vi "record_tsv_LCWFM.vi"(7 "record_on":bool=TRUE, 8 "value_array":dbl[](array[numeric])=[0.0], 10 "time":timestamp, 11 "file_name":string="record") -> (0 "status":bool)   [LabVIEW 2019]
uses:
  <vilib>/Utility/file.llb/Write Delimited Spreadsheet (string).vi
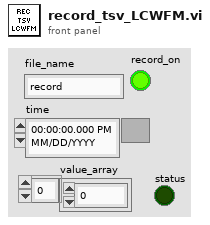
[diagram p1: front panel]
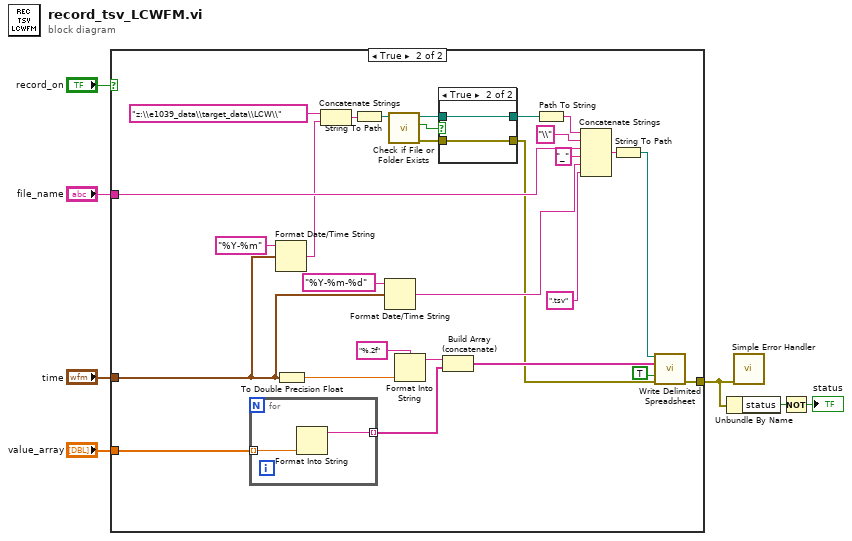
[diagram p0: block diagram]
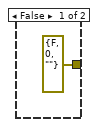
[diagram p2: hidden frame]
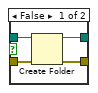
[diagram p3: hidden frame]
diagram:
  n1 = case shown="True" "record_on" {
    tunnel: "file_name" -> [_ w31]
    tunnel: "value_array" -> [_ w20]
    tunnel: "time" -> [_ w18]
    tunnel: [errorcluster {"status"=FALSE, "code"=0, "source"=""} ("error out") w9] -> w3
    frame False {
    }
    frame True {
      n2 = for {
        tunnel: [w38] -> w21 mode=indexing
        tunnel: w20 -> [w37] mode=indexing
        n3 = Format Into String(w37) -> (resulting string=w38:string)  [unwired: 3 in, 1 out]
      }
      n4 = Format Date/Time String(time format string (%c)="%Y-%m", seconds (now)=w18) -> (date/time string=w12:string)  [unwired: 1 in]
      n5 = To Double Precision Float(number=w18) -> (double precision float=w23:dbl)
      n6 = Concatenate Strings("z:\\e1039_data\\target_data\\LCW\\", w12) -> (w33:string)
      n7 = String To Path(string=w33) -> (path=w29:path)
      n8 = Format Date/Time String(time format string (%c)="%Y-%m-%d", seconds (now)=w18) -> (date/time string=w15:string)  [unwired: 1 in]
      n9 = call <vilib>:"Check if File or Folder Exists.vi"("path"=w29) -> ("error out"=w11:errorcluster, "file or folder exists?"=w28:bool, "dup path"=w26:path)  [unwired: 8 in]
      n10 = Format Into String(format string="%.2f", w23) -> (resulting string=w36:string)  [unwired: 2 in, 1 out]
      n11 = case shown="True" w28 {
        tunnel: w26 -> [w42 w44]
        tunnel: [w41 w44] -> w27
        tunnel: w11 -> [w40 w43]
        tunnel: [w39 w43] -> w10
        frame False {
          n12 = Create Folder(path (use dialog)=w42, error in=w40) -> (created path=w41:path, error out=w39:errorcluster)  [unwired: 1 in, 1 out]
        }
        frame True {
        }
      }
      n13 = Build Array (concatenate)(w36, w21) -> (w35:string[])
      n14 = Path To String(path=w27) -> (string=w25:string)
      n15 = Concatenate Strings(w25, "\\", w31, "_" ("string"), w15, ".tsv" ("string")) -> (w30:string)
      n16 = String To Path(string=w30) -> (path=w24:path)
      n17 = call-poly <vilib>:"Write Delimited Spreadsheet.vi"("file path (dialog if empty)"=w24, "1D data"=w35, "append to file? (new file:F)"=TRUE, "error in (no error)"=w10) -> ("error out"=w9:errorcluster)  [unwired: 10 in, 1 out]
    }
  }
  n18 = Unbundle By Name(w3) -> ("status"=w2:bool)
  n19 = call <vilib>:"Simple Error Handler.vi"("error in (no error)"=w3) -> ()  [unwired: 4 in, 5 out]
  n20 = Not(x=w2) -> (.not. x?=→"status":bool)
